vi "Insert (key-value).vi"(8 "error in (no error)":errorcluster, 9 "Value":refnum<class "Generic Plugin.lvclass">, 10 "Key":string, 11 "Parameter to Hardware Map in":refnum<class "Parameter to Hardware Map.lvclass">) -> (0 "error out":errorcluster, 3 "Parameter to Hardware Map out":refnum<class "Parameter to Hardware Map.lvclass">)   [LabVIEW 2020, in "RxnRover.lvlib" / "Parameter to Hardware Map.lvclass"]
doc: "Create and insert a key-value pair into the map using the given key and value."
uses:
  Parameter to Hardware Map.lvclass
  Controller/Generic Plugin.lvclass
  Pair.ctl
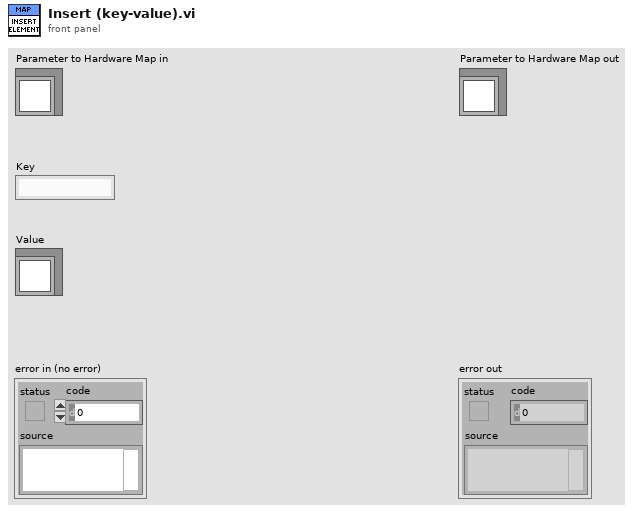
[diagram p1: front panel]
types:
  T1 = typedef "RxnRover.lvlib/Parameter to Hardware Map.lvclass/Pair.ctl" = cluster{"key":string, "values":refnum<class "Generic Plugin.lvclass">[]}
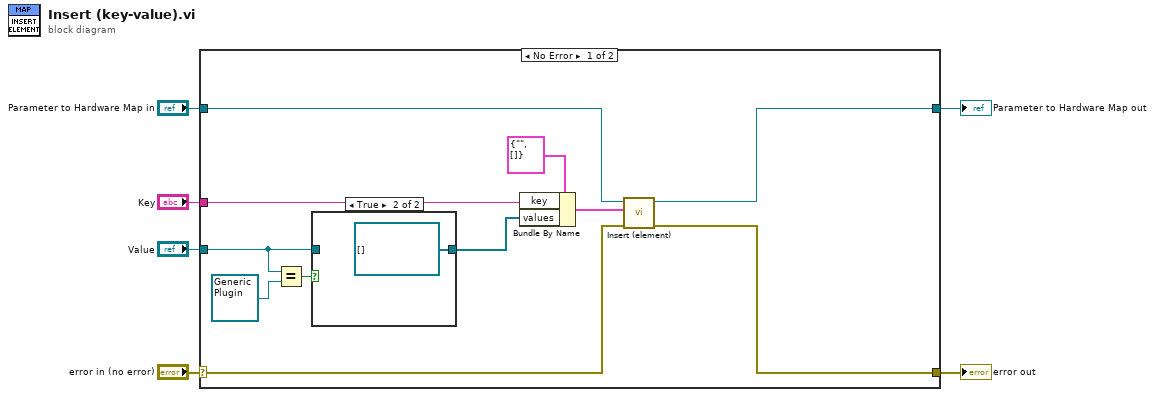
[diagram p0: block diagram]
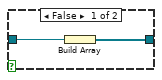
[diagram p2: hidden frame]
diagram:
  n1 = case shown="No Error" "error in (no error)" {
    selector: "error in (no error)" -> [w14 w22]
    tunnel: [w11 w22] -> w5
    tunnel: [w12 w21] -> w3
    tunnel: "Parameter to Hardware Map in" -> [w15 w21]
    tunnel: "Key" -> [w16 _]
    tunnel: "Value" -> [w8 _]
    frame No Error {
      n2 = Equal?(x=w8, y=refnum<class "Generic Plugin.lvclass"> refnum ("Value")) -> (x = y?=w9:bool)
      n3 = case shown="True" w9 {
        tunnel: w8 -> [w19 _]
        tunnel: [w18 refnum<class "Generic Plugin.lvclass">[] []] -> w7
        frame False {
          n4 = Build Array(w19) -> (w18:refnum<class "Generic Plugin.lvclass">[])
        }
        frame True {
        }
      }
      n5 = Bundle By Name(cluster=T1 {"key"="", "values"=[]} ("Key-Value Pair"), "key"=w16, "values"=w7) -> (w13:T1)
      n6 = call "Insert (element).vi"("error in (no error)"=w14, "Key-Value Pair"=w13, "Parameter to Hardware Map in"=w15) -> ("error out"=w11:errorcluster, "Parameter to Hardware Map out"=w12:refnum<class "Parameter to Hardware Map.lvclass">)  [unwired: 7 in]
    }
    frame Error {
    }
  }
  "error out" <- w5
  "Parameter to Hardware Map out" <- w3
